vi "test_of_fixed_array_blocks.vi"() -> ()   [LabVIEW 2009]
panel:
  out "Time 2":u32
  out "Time":u32
  out "element":u8
  out "output array":u8[](array[numeric])
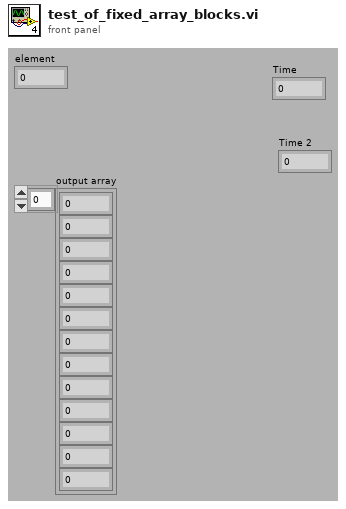
[diagram p1: front panel]
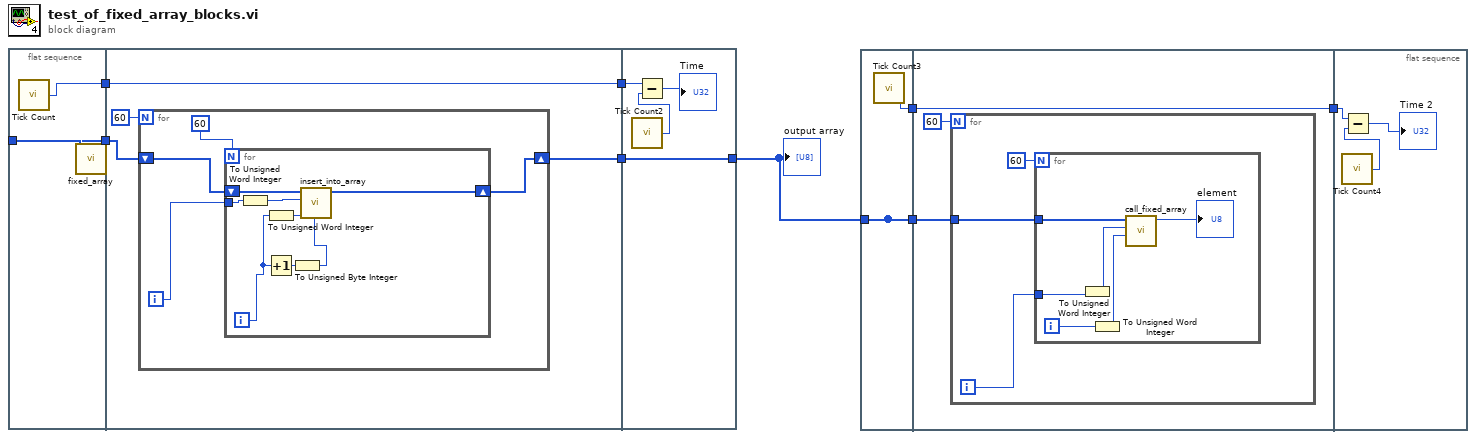
[diagram p0: block diagram]
diagram:
  n1 = flat-sequence {
    tunnel: w9 -> [w11]
    tunnel: [w11] -> w8
    tunnel: [w10] -> w6
    tunnel: w8 -> [w13]
    tunnel: [w14] -> w7
    tunnel: w6 -> [w12]
    tunnel: [w12] -> w5
    tunnel: [w31] -> w1
    tunnel: w7 -> [w31]
    tunnel: w5 -> [w29]
    frame #0 {
      n2 = call "Tick Count"() -> ("Tick Count(Ticks)"=w10:u32)
    }
    frame #1 {
      n3 = for {
        N: 60 -> [_]
        shift-right: [w17] -> w14
        shift-left: w13 -> [w16]
        i -> [w18]
        n4 = for {
          N: 60 -> [_]
          tunnel: w18 -> [w27]
          shift-right: [w25] -> w17
          shift-left: w16 -> [w26]
          i -> [w24]
          n5 = To Unsigned Word Integer(number=w27) -> (unsigned 16bit integer=w20:u16)
          n6 = To Unsigned Word Integer(number=w24) -> (unsigned 16bit integer=w23:u16)
          n7 = Increment(x=w24) -> (x+1=w22:i32)
          n8 = To Unsigned Byte Integer(number=w22) -> (unsigned 8bit integer=w21:u8)
          n9 = call "insert_into_array.vi"("new element/subarray"=w21, "column"=w23, "row"=w20, "array"=w26) -> ("output array"=w25:u8[])  [unwired: 7 in]
        }
      }
    }
    frame #2 {
      n10 = call "Tick Count2"() -> ("Tick Count(Ticks)"=w30:u32)
      n11 = Subtract(x=w29, y=w30) -> (x-y=→"Time":u32)
    }
  }
  n12 = call "fixed_array.vi"() -> ("Array"=w9:u8[])  [unwired: 11 in]
  n13 = flat-sequence {
    tunnel: [w32] -> _
    tunnel: [w32] -> w4
    tunnel: [w33] -> w3
    tunnel: w1 -> [w32]
    tunnel: w4 -> [w35]
    tunnel: w3 -> [w34]
    tunnel: [w34] -> w2
    tunnel: w2 -> [w46]
    frame #0 {
      n14 = call "Tick Count3"() -> ("Tick Count(Ticks)"=w33:u32)
    }
    frame #1 {
      n15 = for {
        N: 60 -> [_]
        tunnel: w35 -> [w37]
        i -> [w38]
        n16 = for {
          N: 60 -> [_]
          tunnel: w38 -> [w45]
          tunnel: w37 -> [w43]
          i -> [w44]
          n17 = To Unsigned Word Integer(number=w45) -> (unsigned 16bit integer=w41:u16)
          n18 = To Unsigned Word Integer(number=w44) -> (unsigned 16bit integer=w40:u16)
          n19 = call "call_fixed_array.vi"("column"=w40, "row"=w41, "array"=w43) -> ("element"=→"element":u8)  [unwired: 8 in]
        }
      }
    }
    frame #2 {
      n20 = call "Tick Count4"() -> ("Tick Count(Ticks)"=w48:u32)
      n21 = Subtract(x=w46, y=w48) -> (x-y=→"Time 2":u32)
    }
  }
  "output array" <- w1
